vi "Blink 5.vi"(8 "Error In":errorcluster) -> (0 "Error Out":errorcluster)   [LabVIEW 2014]
uses:
  <vilib>/Aledyne-TSXperts/Arduino Compatible Compiler for LabVIEW/addons/Arduino SoftwareSerial Wrapper/Arduino SoftwareSerial Wrapper.lvlib
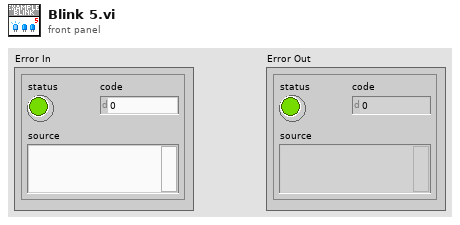
[diagram p1: front panel]
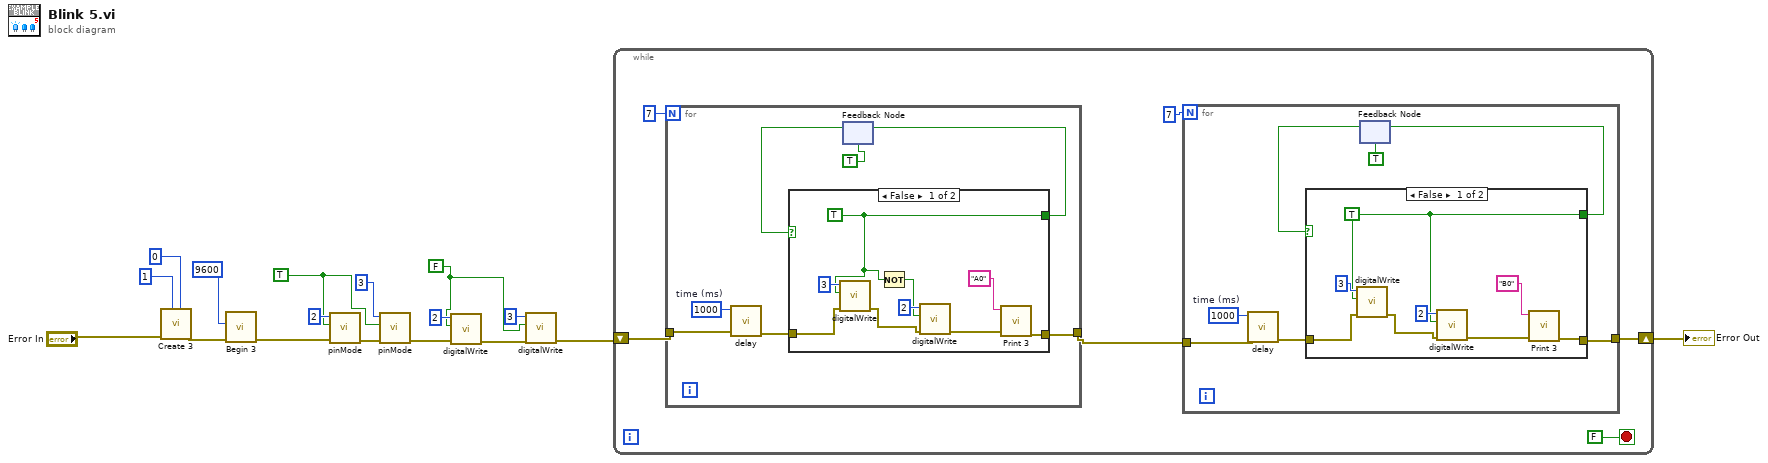
[diagram p0: block diagram]
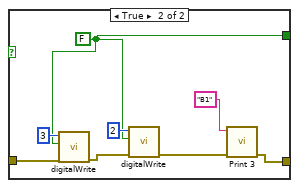
[diagram p2: hidden frame]
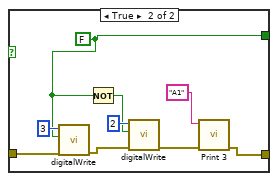
[diagram p3: hidden frame]
diagram:
  w7 = FALSE
  w14 = TRUE
  n1 = call <vilib>:"Create 3.vi"("arduino RX pin"=u8 0, "arduino TX pin"=u8 1, "Error In"="Error In") -> ("Error Out"=w4:errorcluster)  [unwired: 8 in]
  n2 = call <vilib>:"Begin 3.vi"("Error In"=w4, "Baudrate"=u16 9600) -> ("Error Out"=w2:errorcluster)  [unwired: 8 in]
  n3 = call "pinMode.vi"("Error In"=w2, "output?"=w14, "pin number"=2) -> ("Error Out"=w17:errorcluster)  [unwired: 8 in]
  n4 = call "pinMode.vi"("Error In"=w17, "output?"=w14, "pin number"=3) -> ("Error Out"=w10:errorcluster)  [unwired: 8 in]
  n5 = call "digitalWrite.vi"("Error In"=w10, "value"=w7, "pin number"=2) -> ("Error Out"=w9:errorcluster)  [unwired: 8 in]
  n6 = call "digitalWrite.vi"("Error In"=w9, "value"=w7, "pin number"=3) -> ("Error Out"=w8:errorcluster)  [unwired: 8 in]
  n7 = while {
    shift-right: [w20] -> w13
    shift-left: w8 -> [w23]
    stop <- FALSE stop-if-true
    n8 = for {
      N: 7 -> [_]
      tunnel: w23 -> [w53]
      tunnel: [w50] -> w18
      w51 = 1000  # time (ms)
      n9 = call "delay.vi"("Error In"=w53, "time (ms)"=w51) -> ("Error Out"=w52:errorcluster)  [unwired: 9 in]
      n10 = feedback #1(TRUE) -> (w48:bool)
      n11 = case shown="False" w48 {
        tunnel: w52 -> [w61 w71]
        tunnel: [w54 w64] -> w50
        tunnel: [w58 w67] -> w49
        frame False {
          w58 = TRUE
          n12 = call "digitalWrite.vi"("Error In"=w61, "value"=w58, "pin number"=3) -> ("Error Out"=w57:errorcluster)  [unwired: 8 in]
          n13 = Not(x=w58) -> (.not. x?=w59:bool)
          n14 = call "digitalWrite.vi"("Error In"=w57, "value"=w59, "pin number"=2) -> ("Error Out"=w55:errorcluster)  [unwired: 8 in]
          n15 = call <vilib>:"Print 3.vi"("Error In"=w55, "String to print"="A0") -> ("Error Out"=w54:errorcluster)  [unwired: 9 in]
        }
        frame True {
          w67 = FALSE
          n16 = call "digitalWrite.vi"("Error In"=w71, "value"=w67, "pin number"=3) -> ("Error Out"=w68:errorcluster)  [unwired: 8 in]
          n17 = Not(x=w67) -> (.not. x?=w66:bool)
          n18 = call "digitalWrite.vi"("Error In"=w68, "value"=w66, "pin number"=2) -> ("Error Out"=w65:errorcluster)  [unwired: 8 in]
          n19 = call <vilib>:"Print 3.vi"("Error In"=w65, "String to print"="A1") -> ("Error Out"=w64:errorcluster)  [unwired: 9 in]
        }
      }
      n20 = feedback-in #1(w49) -> ()
    }
    n21 = for {
      N: 7 -> [_]
      tunnel: [w28] -> w20
      tunnel: w18 -> [w24]
      w29 = 1000  # time (ms)
      n22 = call "delay.vi"("Error In"=w24, "time (ms)"=w29) -> ("Error Out"=w30:errorcluster)  [unwired: 9 in]
      n23 = feedback #2(TRUE) -> (w26:bool)
      n24 = case shown="False" w26 {
        tunnel: w30 -> [w37 w46]
        tunnel: [w31 w39] -> w28
        tunnel: [w35 w42] -> w27
        frame False {
          w35 = TRUE
          n25 = call "digitalWrite.vi"("Error In"=w37, "value"=w35, "pin number"=3) -> ("Error Out"=w34:errorcluster)  [unwired: 8 in]
          n26 = call "digitalWrite.vi"("Error In"=w34, "value"=w35, "pin number"=2) -> ("Error Out"=w32:errorcluster)  [unwired: 8 in]
          n27 = call <vilib>:"Print 3.vi"("Error In"=w32, "String to print"="B0") -> ("Error Out"=w31:errorcluster)  [unwired: 9 in]
        }
        frame True {
          w42 = FALSE
          n28 = call "digitalWrite.vi"("Error In"=w46, "value"=w42, "pin number"=3) -> ("Error Out"=w43:errorcluster)  [unwired: 8 in]
          n29 = call "digitalWrite.vi"("Error In"=w43, "value"=w42, "pin number"=2) -> ("Error Out"=w40:errorcluster)  [unwired: 8 in]
          n30 = call <vilib>:"Print 3.vi"("Error In"=w40, "String to print"="B1") -> ("Error Out"=w39:errorcluster)  [unwired: 9 in]
        }
      }
      n31 = feedback-in #2(w27) -> ()
    }
  }
  "Error Out" <- w13
